vi "Read State.vi"(8 "error in (no error)":errorcluster, 11 "DefendAreaTacticVSS in":refnum<class "DefendAreaTacticVSS.lvclass">) -> (0 "error out":errorcluster, 2 "State":enum16{"Exit", "Kick", "DefBallPos", "GoToBall"}(ring), 3 "DefendAreaTacticVSS out":refnum<class "DefendAreaTacticVSS.lvclass">)   [LabVIEW 2020, in "DefendAreaTacticVSS.lvclass"]
uses:
  DefendAreaTacticVSS.lvclass
  DefendAreaTacticVSS.lvclass/DefendAreaTacticVSS.ctl
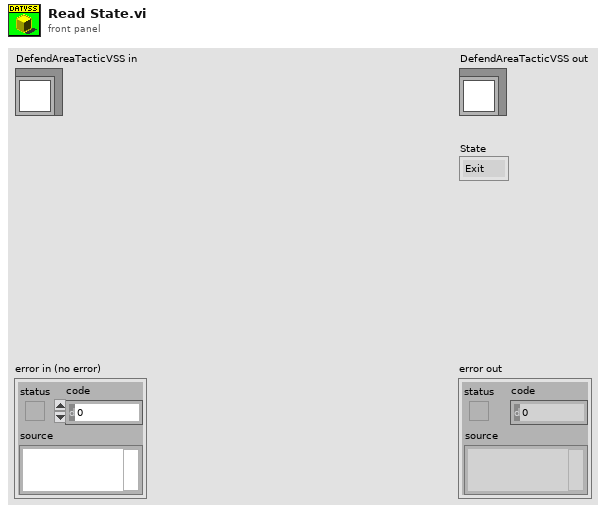
[diagram p1: front panel]
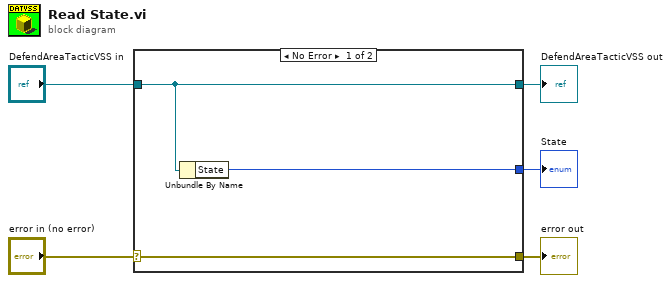
[diagram p0: block diagram]
diagram:
  n1 = case shown="No Error" "error in (no error)" {
    selector: "error in (no error)" -> [w8 w9]
    tunnel: [w8 w9] -> w4
    tunnel: [w7 w10] -> w2
    tunnel: "DefendAreaTacticVSS in" -> [w7 w10]
    tunnel: [w6 _] -> w1
    frame No Error {
      n2 = Unbundle By Name(w7) -> ("State"=w6:enum16{"Exit", "Kick", "DefBallPos", "GoToBall"})
    }
    frame Error {
    }
  }
  "error out" <- w4
  "DefendAreaTacticVSS out" <- w2
  "State" <- w1
